vi "FOR Challenge.vi"() -> ()   [LabVIEW 2014]
panel:
  out "Counter value":i32
  in  "Count until number":i32
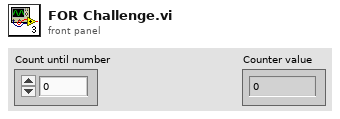
[diagram p1: front panel]
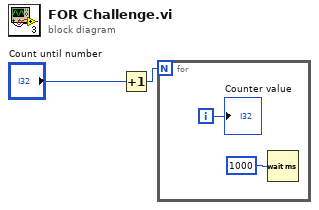
[diagram p0: block diagram]
diagram:
  n1 = Increment(x="Count until number") -> (x+1=w1:i32)
  n2 = for {
    N: w1 -> [_]
    i -> [w3]
    n3 = Wait (ms)(milliseconds to wait=u32 1000) -> ()  [unwired: 1 out]
    "Counter value" <- w3
  }
